vi "Set Frequency.vi"(9 "test signal\nfreq (Hz)":dbl=100000.0 format="%.3e", 11 "GPIB addess":string="17") -> ()   [LabVIEW 2015, in "HP4192A IA.lvclass"]
uses:
  HP4192A IA.lvclass
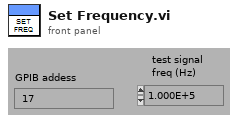
[diagram p1: front panel]
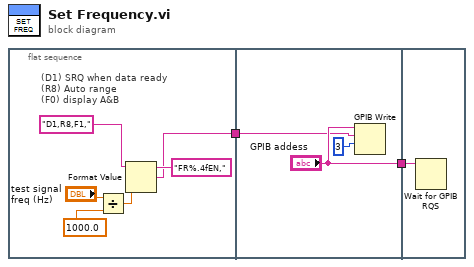
[diagram p0: block diagram]
diagram:
  n1 = flat-sequence {
    tunnel: [w3] -> w1
    tunnel: ["GPIB addess"] -> w2
    tunnel: w1 -> [w9]
    tunnel: w2 -> [w12]
    frame #0 {
      # "(D1) SRQ when data ready\n(R8) Auto range\n(F0) display A&B"
      n2 = Divide(x="test signal\nfreq (Hz)", y=1000.0) -> (x/y=w7:dbl)
      n3 = Format Value(string ("")="D1,R8,F1,", format string="FR%.4fEN,", value (0)=w7) -> (output string=w3:string)
    }
    frame #1 {
      n4 = GPIB Write(0:"GPIB addess", 1:w9, 2:3) -> ()  [unwired: 2 in, 2 out]
    }
    frame #2 {
      n5 = Wait for GPIB RQS(4:w12) -> ()  [unwired: 2 in, 2 out]
    }
  }
